vi "Simple Sound.vi"(5 "Action":enum16{"Open", "Write", "Close"}(ring)=enum."Write", 6 "error in":errorcluster, 7 "sound format":T2={"sample rate (S/s)"=44100.0, "number of channels"=1, "bits per sample"=16}, 8 "task ID":T1 format="%.0x", 9 "data":waveform(dbl)={"t0"=timestamp(0 s since 1904-01-01), "dt"=0.0, "Y"=[0.0]}) -> (0 "error out":errorcluster={"status"=TRUE, "code"=4801, "source"="Sound Output Write (DBL).vi->Sound Output Write (DBL Single).vi->Simple Sound.vi\r\n"}, 2 "task ID out":T1 format="%.0x", 3 "sample rate (S/s)":dbl=44100.0)   [LabVIEW 2022 SP3]
uses:
  <vilib>/sound2/lvsound2.llb/Sound Data Format.ctl
  <vilib>/sound2/lvsound2.llb/Sound Output Task ID.ctl
  <vilib>/sound2/lvsound2.llb/Sound Output Write (DBL Single).vi
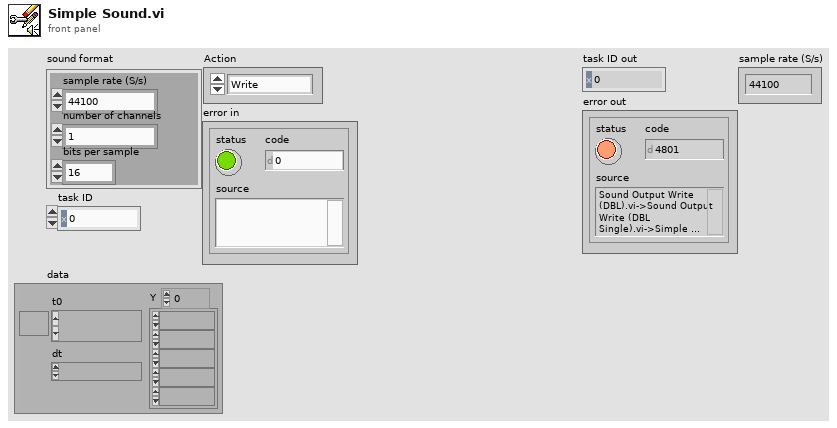
[diagram p1: front panel]
types:
  T1 = typedef "Sound Output Task ID.ctl" = u32
  T2 = typedef "Sound Data Format.ctl" = cluster{"sample rate (S/s)":dbl, "number of channels":i32, "bits per sample":i32}
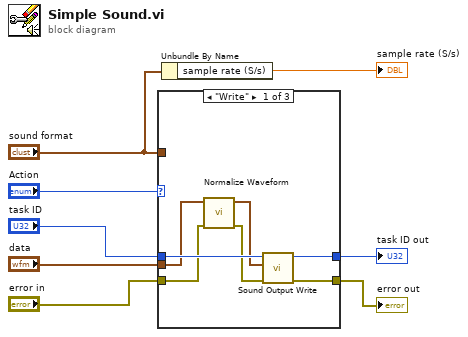
[diagram p0: block diagram]
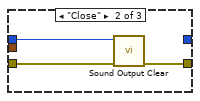
[diagram p2: hidden frame]
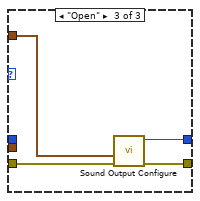
[diagram p3: hidden frame]
diagram:
  n1 = case shown="\"Write\"" "Action" {
    tunnel: "sound format" -> [_ _ w22]
    tunnel: [w15 _ w21] -> w5
    tunnel: "task ID" -> [w14 w17 _]
    tunnel: "data" -> [w11 _ _]
    tunnel: [w13 w18 w20] -> w4
    tunnel: "error in" -> [w10 w16 w19]
    frame "Write" {
      n2 = call <vilib>:"Normalize Waveform.vi"("error in (no error)"=w10, "waveform in"=w11) -> ("error out"=w9:errorcluster, "normalized waveform"=w12:waveform(dbl))  [unwired: 6 in, 2 out]
      n3 = call-poly <vilib>:"Sound Output Write.vi"("error in (no error)"=w9, "data"=w12, "task ID"=w14) -> ("error out"=w13:errorcluster, "task ID out"=w15:T1)  [unwired: 7 in]
    }
    frame "Close" {
      n4 = call <vilib>:"Sound Output Clear.vi"("error in (no error)"=w16, "task ID"=w17) -> ("error out"=w18:errorcluster)  [unwired: 9 in]
    }
    frame "Open" {
      n5 = call <vilib>:"Sound Output Configure.vi"("error in (no error)"=w19, "sound format"=w22) -> ("error out"=w20:errorcluster, "task ID"=w21:T1)  [unwired: 8 in]
    }
  }
  "task ID out" <- w5
  "error out" <- w4
  n6 = Unbundle By Name "Unbundle By Name"("sound format") -> ("sample rate (S/s)"=→"sample rate (S/s)":dbl)
